vi "Wizard Save Library.vi"(8 "error in (no error)":errorcluster, 9 "Lib Full Path":path, 10 "Library in":refnum<vi>, 11 "Project in":refnum<vi>) -> (0 "error out":errorcluster)   [LabVIEW 2014]
doc: "<B>Copyright</B>: (c) 2015 MHWirth. All rights reserved.\n\nThis subVI saves the library in the given path, and closes the project.\n\nNot available in Run-time Engine."
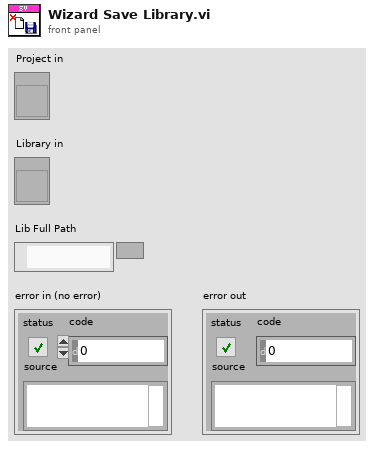
[diagram p1: front panel]
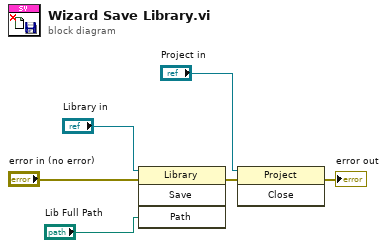
[diagram p0: block diagram]
diagram:
  n1 = invoke class="Library" method="Save"(reference="Library in", error in="error in (no error)", "Path"="Lib Full Path") -> (error out=w4:errorcluster)  [unwired: 1 in, 3 out]
  n2 = invoke class="Project" method="Close"(reference="Project in", error in=w4) -> (error out=→"error out":errorcluster)  [unwired: 1 in, 2 out]
